vi "Create Error.vi"(1 "Show call chain?":bool, 2 "Error Message Type":T1, 3 "Error iteration number (i)":i32) -> (0 "Error Out":errorcluster)   [LabVIEW 2016, in "Anti-Spam Tester (AST).lvlib"]
doc: "Blank VI with error handling."
uses:
  Anti-Spam Tester (AST).lvlib
  Spam Error Message Type (enum).ctl
panel:
  # "Input\nInputs to the VI"
  # "Development\nControls or indicators that are useful for development or testing, but which are not outputs of the VI."
  # "Output\nOutputs of the VI"
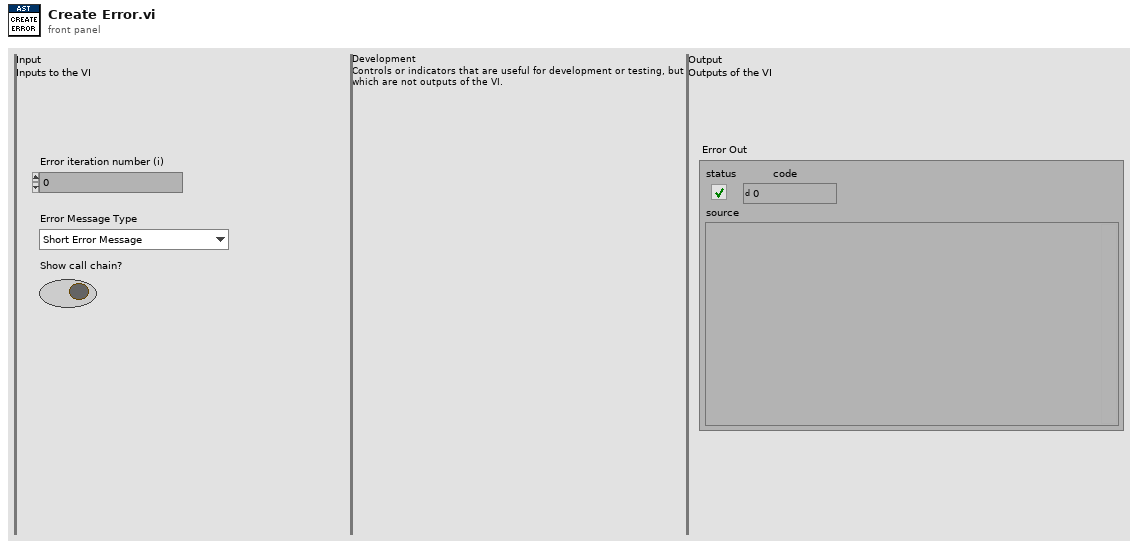
[diagram p1: front panel]
types:
  T1 = typedef "Anti-Spam Tester (AST).lvlib/Spam Error Message Type (enum).ctl" = enum16{"Short Error Message", "Long Error Message"}
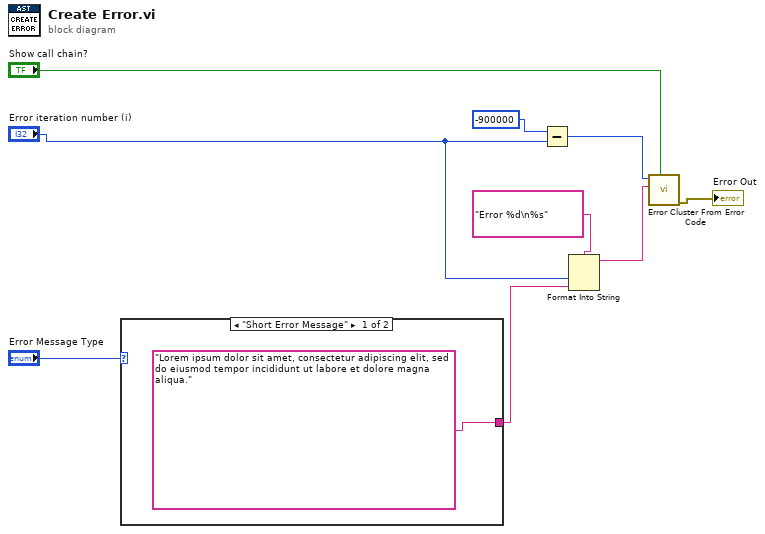
[diagram p0: block diagram]
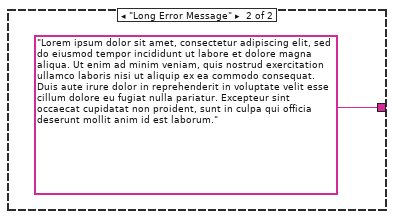
[diagram p2: hidden frame]
diagram:
  n1 = case shown="\"Short Error Message\"" "Error Message Type" {
    tunnel: ["Lorem ipsum dolor sit amet, consectetur adipiscing elit, sed do eiusmod tempor incididunt ut labore et dolore magna aliqua." "Lorem ipsum dolor sit amet, consectetur adipiscing elit, sed do eiusmod tempor incididunt ut labore et dolore magna aliqua. Ut enim ad minim veniam, quis nostrud exercitation ullamco laboris nisi ut aliquip ex ea commodo consequat. Duis aute irure dolor in reprehenderit in voluptate velit esse cillum dolore eu fugiat nulla pariatur. Excepteur sint occaecat cupidatat non proident, sunt in culpa qui officia deserunt mollit anim id est laborum."] -> w3
    frame "Short Error Message" {
    }
    frame "Long Error Message" {
    }
  }
  n2 = Subtract(x=-900000, y="Error iteration number (i)") -> (x-y=w8:i32)
  n3 = Format Into String(format string="Error %d\n%s", "Error iteration number (i)", w3) -> (resulting string=w5:string)  [unwired: 2 in, 1 out]
  n4 = call <vilib>:"Error Cluster From Error Code.vi"("show call chain? (False)"="Show call chain?", "error message (\"\")"=w5, "error code (0)"=w8) -> ("error out"=→"Error Out":errorcluster)  [unwired: 6 in]
